vi "Validate Get Connections Inputs.vi"(6 "site":i32, 8 "error in":errorcluster, 9 "instrument type id":string, 10 "pin or relay names":string[](array[string]), 11 "connection map":refnum<class "Connection Map.lvclass">) -> (0 "error out":errorcluster, 3 "connection map out":refnum<class "Connection Map.lvclass">)   [LabVIEW 2020, in "NI Session Management V1 Client.lvlib" / "Session Reservation.lvclass"]
uses:
  Session Reservation.lvclass
  Connection Map/Connection Map.lvclass
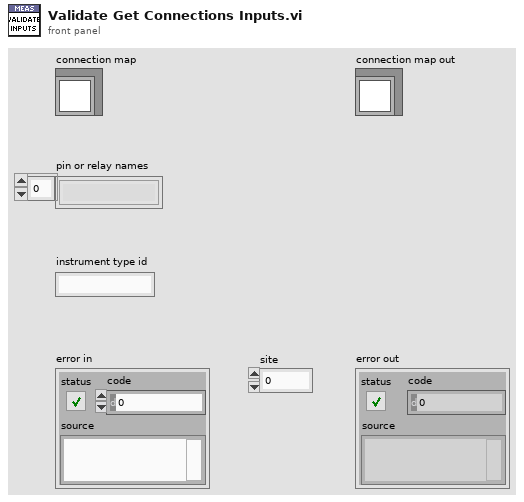
[diagram p1: front panel]
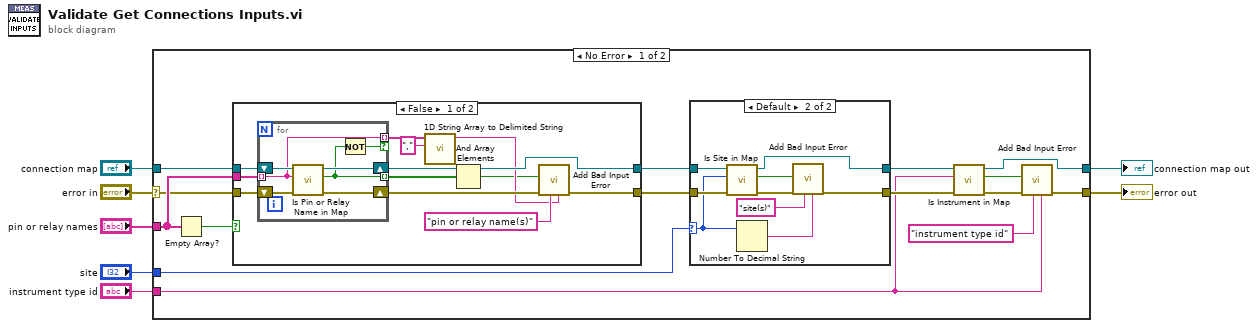
[diagram p0: block diagram]
diagram:
  n1 = case shown="No Error" "error in" {
    selector: "error in" -> [w18 w56]
    tunnel: "pin or relay names" -> [w21 _]
    tunnel: "site" -> [w22 _]
    tunnel: "instrument type id" -> [w9 _]
    tunnel: "connection map" -> [w19 w55]
    tunnel: [w11 w56] -> w2
    tunnel: [w13 w55] -> w1
    frame No Error {
      n2 = Empty Array?(array=w21) -> (empty?=w20:bool)
      n3 = case shown="False" w20 {
        tunnel: w18 -> [w34 w43]
        tunnel: w19 -> [w33 w42]
        tunnel: [w29 w43] -> w16
        tunnel: [w32 w42] -> w17
        tunnel: w21 -> [w31 _]
        frame False {
          n4 = for {
            tunnel: w31 -> [w37] mode=indexing
            shift-right: [w38] -> w30
            shift-left: w34 -> [w41]
            shift-right: [w39] -> w32
            shift-left: w33 -> [w40]
            tunnel: [w37] -> w27 mode=indexing if=w36
            tunnel: [w35] -> w24 mode=indexing
            n5 = call "Is Pin or Relay Name in Map.vi"("error in"=w41, "pin or relay name"=w37, "connection map in"=w40) -> ("error out"=w38:errorcluster, "pin or relay name in map"=w35:bool, "connection map out"=w39:refnum<class "Connection Map.lvclass">)  [unwired: 6 in]
            n6 = Not(x=w35) -> (.not. x?=w36:bool)
          }
          n7 = call <vilib>:"1D String Array to Delimited String.vi"("delimiter"=",", "string array"=w27) -> ("delimited string"=w25:string)  [unwired: 9 in]
          n8 = And Array Elements(Boolean array=w24) -> (logical AND=w23:bool)
          n9 = call "Add Bad Input Error.vi"("missing value"=w25, "name"="pin or relay name(s)", "error in"=w30, "in connections map"=w23) -> ("error out"=w29:errorcluster)  [unwired: 7 in]
        }
        frame True {
        }
      }
      n10 = case shown="Default" w22 {
        selector: w22 -> [_ w49]
        tunnel: w16 -> [w44 w54]
        tunnel: w17 -> [w45 w53]
        tunnel: [w44 w51] -> w15
        tunnel: [w45 w52] -> w14
        frame -1 {
        }
        frame Default {
          n11 = call "Is Site in Map.vi"("error in"=w54, "site"=w49, "connection map in"=w53) -> ("error out"=w50:errorcluster, "site in map"=w46:bool, "connection map out"=w52:refnum<class "Connection Map.lvclass">)  [unwired: 6 in]
          n12 = Number To Decimal String(number=w49) -> (decimal integer string=w48:string)  [unwired: 1 in]
          n13 = call "Add Bad Input Error.vi"("missing value"=w48, "name"="site(s)" ("String 2"), "error in"=w50, "in connections map"=w46) -> ("error out"=w51:errorcluster)  [unwired: 7 in]
        }
      }
      n14 = call "Is Instrument in Map.vi"("error in"=w15, "instrument type id"=w9, "connection map in"=w14) -> ("error out"=w12:errorcluster, "instrument in map"=w10:bool, "connection map out"=w13:refnum<class "Connection Map.lvclass">)  [unwired: 6 in]
      n15 = call "Add Bad Input Error.vi"("missing value"=w9, "name"="instrument type id", "error in"=w12, "in connections map"=w10) -> ("error out"=w11:errorcluster)  [unwired: 7 in]
    }
    frame Error {
    }
  }
  "error out" <- w2
  "connection map out" <- w1
